vi "niRFUtil WFM Concatenate Waveform Array (real wfm).vi"(1 "Waveform Array In":T1[](array[typedef]) {"y" min=0 max=127 format="%.2f"; "dx" format="%^.2e"; "x0" format="%^.2e"}) -> (0 "Waveform Out":T1 {"y" min=0 max=127 format="%.2f"; "dx" format="%^.2e"; "x0" format="%^.2e"})   [LabVIEW 2015, in "niRFUtil.lvlib"]
doc: "(c) Copyright 2006, National Instruments, Inc. This VI may not be duplicated, sold, or distributed without written consent from National Instruments."
uses:
  niRFUtil.lvlib
  Includes/niRFUtil INC Real Waveform.ctl
  Includes/niRFUtil INC Real Array.ctl
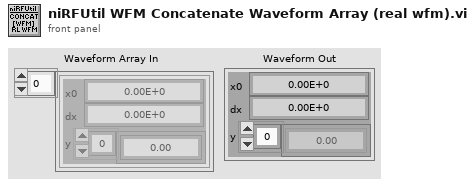
[diagram p1: front panel]
types:
  T1 = typedef "niRFUtil.lvlib/niRFUtil INC Real Waveform.ctl" = cluster{"x0":dbl, "dx":dbl, "y":T2}
  T2 = typedef "niRFUtil.lvlib/niRFUtil INC Real Array.ctl" = sgl[]
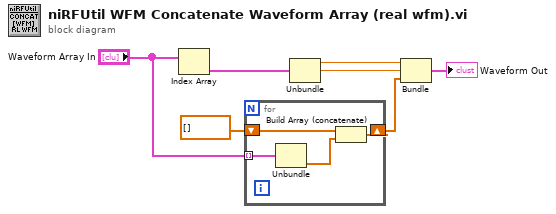
[diagram p0: block diagram]
diagram:
  n1 = Index Array(array="Waveform Array In") -> (element=w4:T1)  [unwired: 1 in]
  n2 = for {
    tunnel: "Waveform Array In" -> [w11] mode=indexing
    shift-right: [w8] -> w2
    shift-left: sgl[] [] ("y") -> [w10]
    n3 = Unbundle(w11) -> ("y"=w9:T2)  [unwired: 2 out]
    n4 = Build Array (concatenate)(w10, w9) -> (w8:T2)
  }
  n5 = Unbundle(w4) -> ("x0"=w7:dbl, "dx"=w6:dbl)  [unwired: 1 out]
  n6 = Bundle("x0"=w7, "dx"=w6, "y"=w2) -> (→"Waveform Out":cluster{"x0":dbl, "dx":dbl, "y":T2})  [unwired: 1 out]
